vi "GetFileNames.vi"(8 "error in (no error)":errorcluster, 11 "path":path) -> (0 "error out":errorcluster, 1 "Files with .json extension":string[](array[string]), 2 "Array":i32[](array[numeric]), 3 "filenames":string[](array[string]))   [LabVIEW 2015]
panel:
  out "String":string
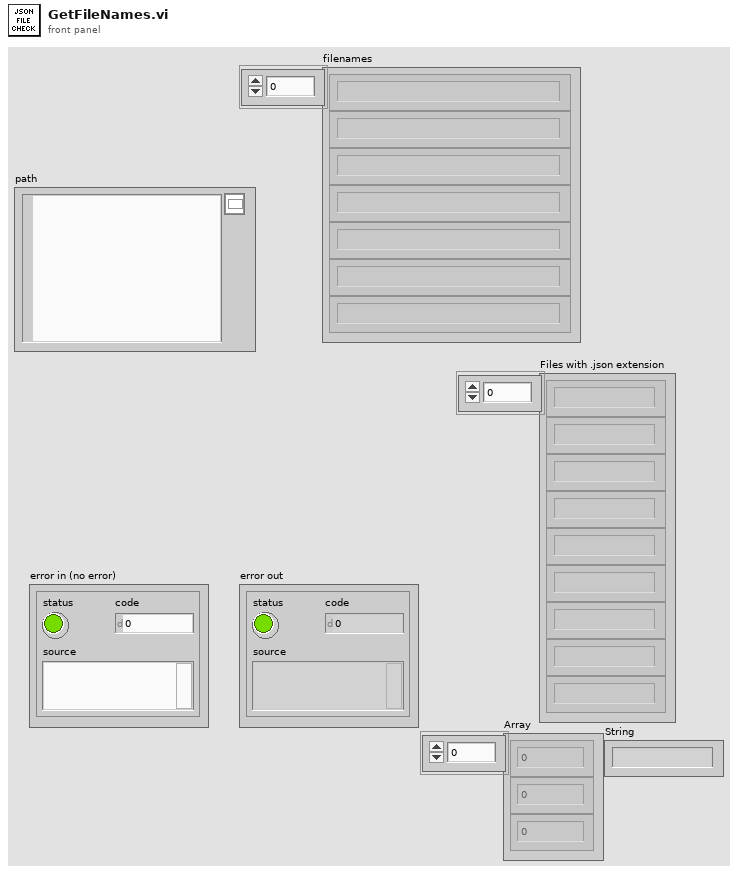
[diagram p1: front panel]
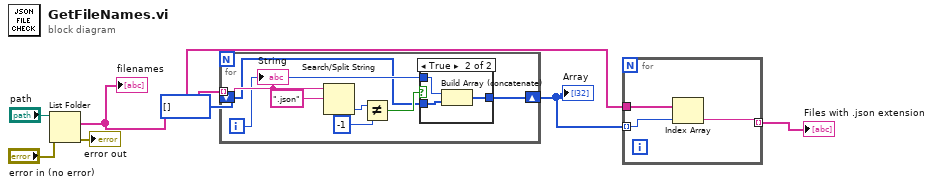
[diagram p0: block diagram]
diagram:
  n1 = List Folder(path="path", error in="error in (no error)") -> (filenames=w4:string[], error out=→"error out":errorcluster)  [unwired: 2 in, 2 out]
  "filenames" <- w4
  n2 = for {
    tunnel: w4 -> [w14] mode=indexing
    shift-right: [w9] -> w3
    shift-left: i32[] [] -> [w8]
    i -> [w10]
    n3 = Search/Split String(string=w14, search string/char (-)=".json" ("regular expression")) -> (offset of match=w13:i32)  [unwired: 1 in, 2 out]
    n4 = Not Equal?(x=w13, y=-1) -> (x != y?=w11:bool)
    n5 = case shown="True" w11 {
      tunnel: w10 -> [_ w19]
      tunnel: [w16 w18] -> w9
      tunnel: w8 -> [w16 w17]
      frame False {
      }
      frame True {
        n6 = Build Array (concatenate)(w19, w17) -> (w18:i32[])
      }
    }
    "String" <- w14
  }
  "Array" <- w3
  n7 = for {
    tunnel: w3 -> [w22] mode=indexing
    tunnel: w4 -> [w21]
    tunnel: [w20] -> w5 mode=indexing
    n8 = Index Array(array=w21, index=w22) -> (element=w20:string)
  }
  "Files with .json extension" <- w5
